vi "GenerateDateString.vi"() -> (0 "String":string)   [LabVIEW 2018]
uses:
  <vilib>/regexp/Match Regular Expression.xnode
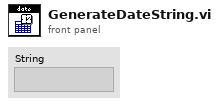
[diagram p1: front panel]
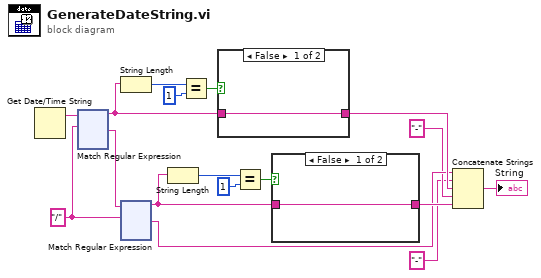
[diagram p0: block diagram]
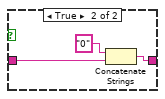
[diagram p2: hidden frame]
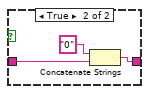
[diagram p3: hidden frame]
diagram:
  w3 = "/" ("regular expression")
  n1 = Get Date/Time String() -> (date string=w1:string)  [unwired: 3 in, 1 out]
  n2 = xnode "Match Regular Expression"("input string"=w1, "regular expression"=w3) -> ("before match"=w10:string, "after match"=w2:string)  [unwired: 4 in, 3 out]
  n3 = String Length(string=w10) -> (length=w7:i32)
  n4 = xnode "Match Regular Expression"("input string"=w2, "regular expression"=w3) -> ("before match"=w15:string, "after match"=w6:string)  [unwired: 4 in, 3 out]
  n5 = String Length(string=w15) -> (length=w14:i32)
  n6 = Equal?(x=w7, y=1) -> (x = y?=w9:bool)
  n7 = case shown="False" w9 {
    tunnel: w10 -> [w18 w21]
    tunnel: [w18 w19] -> w11
    frame False {
    }
    frame True {
      n8 = Concatenate Strings("0" ("string"), w21) -> (w19:string)
    }
  }
  n9 = Equal?(x=w14, y=1) -> (x = y?=w12:bool)
  n10 = case shown="False" w12 {
    tunnel: w15 -> [w22 w25]
    tunnel: [w22 w23] -> w16
    frame False {
    }
    frame True {
      n11 = Concatenate Strings("0" ("string"), w25) -> (w23:string)
    }
  }
  n12 = Concatenate Strings(w6, "-" ("string"), w11, "-" ("string"), w16) -> (→"String":string)
